vi "Send Log Data.vi"(11 "signal in":waveform(dbl)) -> ()   [LabVIEW 2019, in "Adquisiion2.lvlib"]
uses:
  Adquisiion2.lvlib
  <vilib>/measure/matone.llb/Extract Single Tone Information 1 Chan.vi
  <vilib>/measure/mascope.llb/Amplitude and Levels 1 chan.vi
  <vilib>/measure/NI_MAPro.lvlib
  logging/logging.lvlib
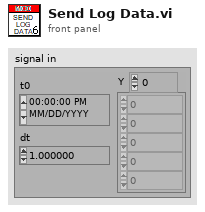
[diagram p1: front panel]
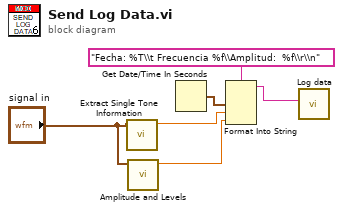
[diagram p0: block diagram]
diagram:
  n1 = call-poly <vilib>:"Extract Single Tone Information.vi"("time signal in"="signal in") -> ("detected frequency"=w5:dbl)  [unwired: 5 in, 5 out]
  n2 = call-poly <vilib>:"Amplitude and Levels.vi"("signal in"="signal in") -> ("amplitude"=w6:dbl)  [unwired: 7 in, 3 out]
  n3 = Get Date/Time In Seconds() -> (seconds since 1Jan1904=w4:timestamp)
  n4 = Format Into String(format string="Fecha: %T\\t Frecuencia %f\\Amplitud:  %f\\r\\n", w4, w5, w6) -> (resulting string=w1:string)  [unwired: 2 in, 1 out]
  n5 = call "Log data.vi"("Log Data"=w1) -> ()  [unwired: 10 in, 1 out]
